vi "74HC153和74HC20设计八选一逻辑电路.vi"() -> ()   [LabVIEW 2018]
panel:
  in  "S2":bool
  in  "S1":bool
  in  "S0":bool
  in  "确定按钮":bool
  out "Y":bool
  in  "D7":bool
  in  "D6":bool
  in  "D5":bool
  in  "D4":bool
  in  "D3":bool
  in  "D2":bool
  in  "D1":bool
  in  "D0":bool
  # "74HC153：双四选一芯片"
  # "74HC20：与非门"
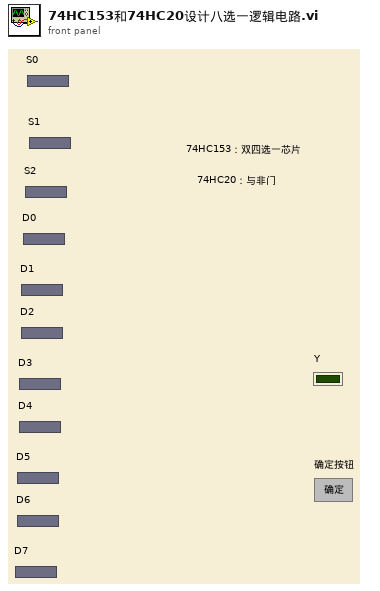
[diagram p1: front panel]
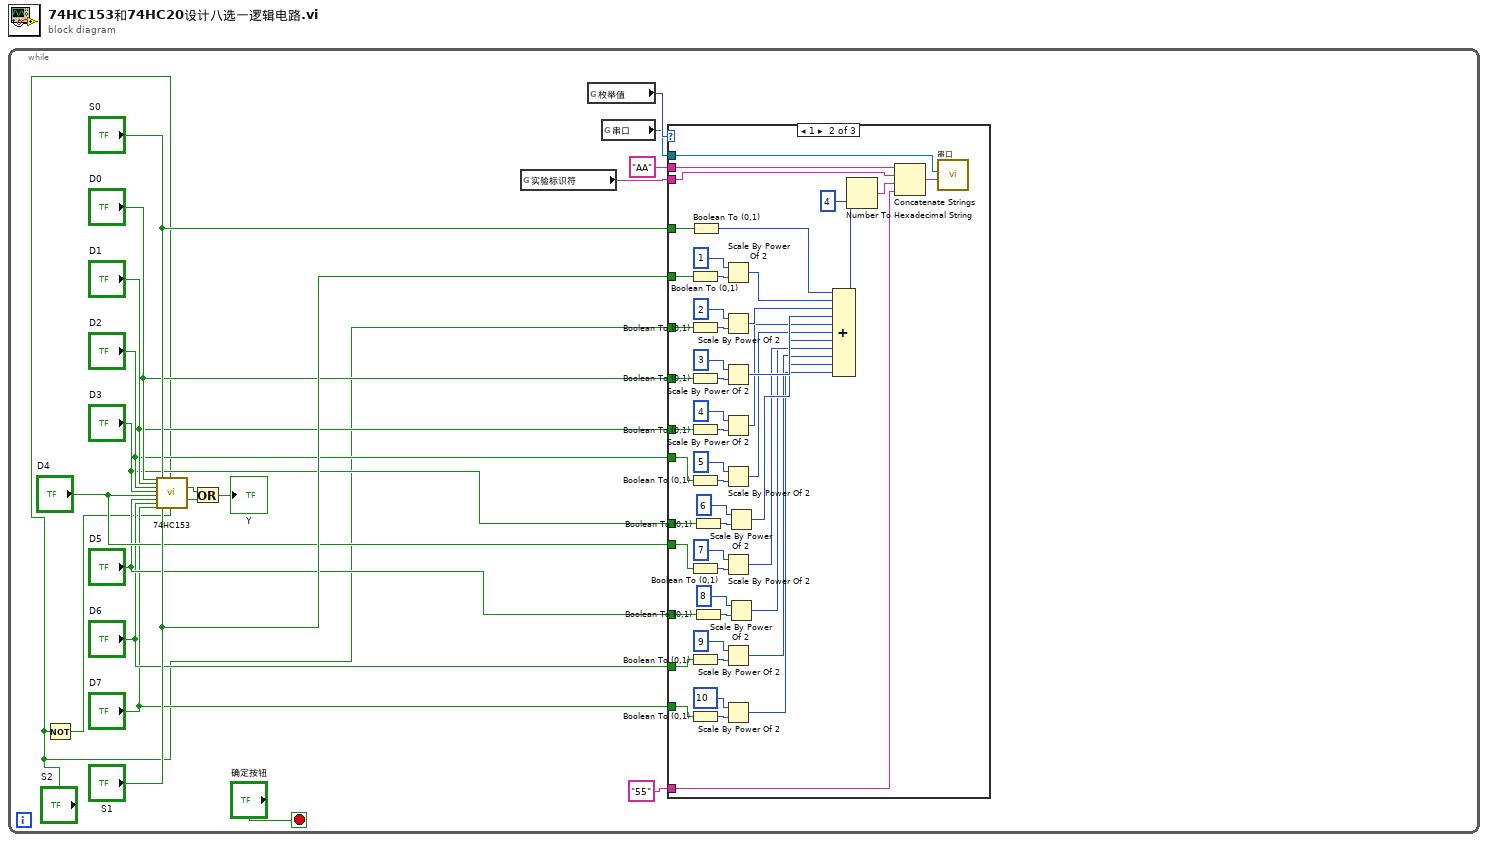
[diagram p0: block diagram]
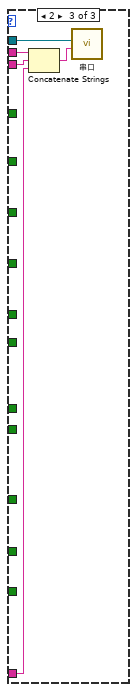
[diagram p3: hidden frame]
diagram:
  n1 = while {
    stop <- "确定按钮" stop-if-true
    n2 = Not(x="S2") -> (.not. x?=w2:bool)
    n3 = call "74HC153.vi"("D10"="D0", "D11"="D1", "D12"="D2", "D13"="D3", "D20"="D4", "D21"="D5", "D22"="D6", "D23"="D7", "S0"="S0", "S1"="S1", "EN1"="S2", "EN2"=w2) -> ("Y1"=w21:bool, "Y2"=w20:bool)  [unwired: 14 in]
    n4 = Or(x=w21, y=w20) -> (x .or. y?=→"Y":bool)
    n5 = global read "全局变量.vi" "实验标识符"() -> (w15:string)
    n6 = global read "全局变量.vi" "枚举值"() -> (w17:i8)
    n7 = global read "全局变量.vi" "串口"() -> (w16:refnum<visa-resource-name>)
    n8 = case shown="1" w17 {
      tunnel: w16 -> [_ w66 w74]
      tunnel: w15 -> [_ w65 w75]
      tunnel: "55" -> [_ w64 w72]
      tunnel: "AA" -> [_ w63 w73]
      tunnel: "S0" -> [_ w32 _]
      tunnel: "S1" -> [_ w31 _]
      tunnel: "S2" -> [_ w30 _]
      tunnel: "D0" -> [_ w29 _]
      tunnel: "D1" -> [_ w28 _]
      tunnel: "D2" -> [_ w27 _]
      tunnel: "D3" -> [_ w26 _]
      tunnel: "D4" -> [_ w25 _]
      tunnel: "D5" -> [_ w24 _]
      tunnel: "D6" -> [_ w23 _]
      tunnel: "D7" -> [_ w22 _]
      frame 0, Default {
      }
      frame 1 {
        n9 = Boolean To (0,1)(Boolean=w31) -> (0, 1=w68:i16)
        n10 = Boolean To (0,1)(Boolean=w30) -> (0, 1=w58:i16)
        n11 = Boolean To (0,1)(Boolean=w29) -> (0, 1=w56:i16)
        n12 = Boolean To (0,1)(Boolean=w28) -> (0, 1=w54:i16)
        n13 = Boolean To (0,1)(Boolean=w27) -> (0, 1=w52:i16)
        n14 = Boolean To (0,1)(Boolean=w25) -> (0, 1=w45:i16)
        n15 = Boolean To (0,1)(Boolean=w23) -> (0, 1=w41:i16)
        n16 = Boolean To (0,1)(Boolean=w22) -> (0, 1=w39:i16)
        n17 = Boolean To (0,1)(Boolean=w32) -> (0, 1=w70:i16)
        n18 = Boolean To (0,1)(Boolean=w26) -> (0, 1=w47:i16)
        n19 = Boolean To (0,1)(Boolean=w24) -> (0, 1=w43:i16)
        n20 = Scale By Power Of 2(n=1, x=w68) -> (x*2^n=w69:i16)
        n21 = Scale By Power Of 2(n=2, x=w58) -> (x*2^n=w59:i16)
        n22 = Scale By Power Of 2(n=3, x=w56) -> (x*2^n=w50:i16)
        n23 = Scale By Power Of 2(n=4, x=w54) -> (x*2^n=w49:i16)
        n24 = Scale By Power Of 2(n=5, x=w52) -> (x*2^n=w48:i16)
        n25 = Scale By Power Of 2(n=7, x=w45) -> (x*2^n=w36:i16)
        n26 = Scale By Power Of 2(n=9, x=w41) -> (x*2^n=w34:i16)
        n27 = Scale By Power Of 2(n=10, x=w39) -> (x*2^n=w33:i16)
        n28 = Scale By Power Of 2(n=6, x=w47) -> (x*2^n=w37:i16)
        n29 = Scale By Power Of 2(n=8, x=w43) -> (x*2^n=w35:i16)
        n30 = Compound Arithmetic op=ADD ("复合运算")(w70, w69, w59, w50, w49, w48, w37, w36, w35, w34, w33) -> (w62:i16)
        n31 = Number To Hexadecimal String(1:4, 2:w62) -> (0:w60:string)
        n32 = Concatenate Strings(w63, w65, w60, w64) -> (w71:string)
        n33 = call "串口.vi"("字符串"=w71, "VISA resource name"=w66) -> ()  [unwired: 10 in]
      }
      frame 2 {
        n34 = Concatenate Strings(w73, w75, w72) -> (w76:string)
        n35 = call "串口.vi"("字符串"=w76, "VISA resource name"=w74) -> ()  [unwired: 10 in]
      }
    }
  }
